vi "time_lua.vi"(5 "LuaVIEW reference":T1) -> (15 "error out":errorcluster)   [LabVIEW 2012]
doc: "Returns the time in seconds since the LabVIEW epoch (1-Jan-1904 00:00:00 GMT). When no parameter is specified, it returns the current time as obtained via \"Library Time.vi\", which exists to allow custom time sources. Its default implementation simply calls \"Get Date/Time In Seconds\" LabVIEW node, which in turn obtains its time from the system clock. Beware that the system clock has a platform dependent resolution and will drift unless corrected for, e.g. using the ntp protocol.\n\nWhen a parameter is specified, it should specify a date/time via a table with the following format: {year=<1904..2040>,month=<1..12>,day=<1..31>,[hour=<0..23>],[min=<0..59>],[sec=<0..59>]}. When the optional hour, min, or sec entries are omitted, they default to zero. The conversion to a time in seconds is performed using the standard \"Date/Time To Seconds\" LabVIEW function.\n\nBEWARE: the \"Date/Time To Seconds\" function yields a result that depends on the timezone and platform. Under Windows, the function corrects for daylight savings, when enabled. Under Linux, it does not, at least for LabVIEW versions 7.0 and 7.1. This is a bug: it yields a numerical time that can be one hour off when displayed via \"Format Date/Time String\".\nParameters:\n[tab:date]\nResults:\nnum:time\nErrors:\nInvalid date table.\nEntry out of range."
uses:
  typedefs/t_LuaVIEW Reference.ctl
  subvis/private/LuaVIEW Push (number).vi
  subvis/private/LuaVIEW Pull (flat data).vi
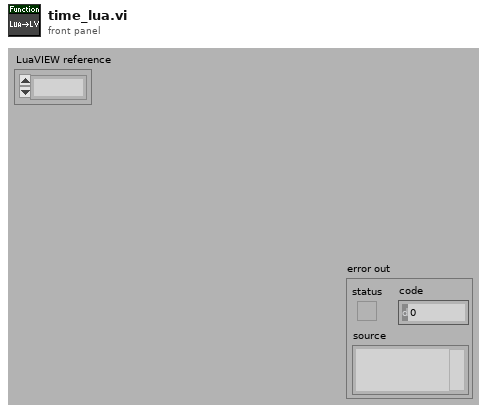
[diagram p1: front panel]
types:
  T1 = typedef "t_LuaVIEW Reference.ctl" = refnum<k1>
  T2 = cluster{"second":i32, "minute":i32, "hour":i32, "day of month":i32, "month":i32, "year":i32, "day of week":i32, "day of year":i32, "is DST":i32}
  T3 = cluster{"year":i32, "month":i32, "day":i32, "hour":i32, "min":i32, "sec":i32}
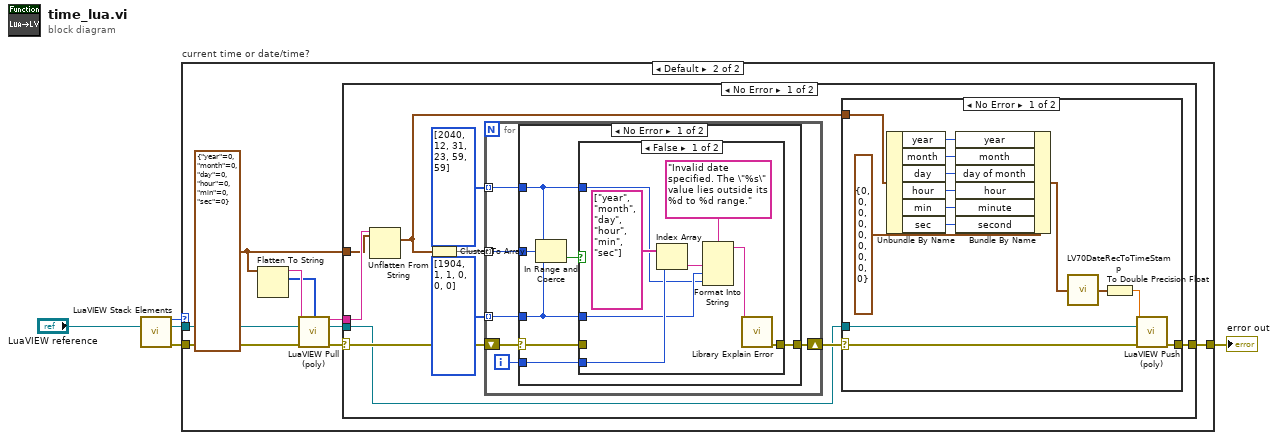
[diagram p0: block diagram]
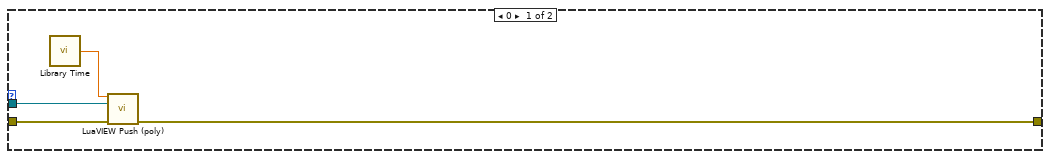
[diagram p2: hidden frame]
diagram:
  n1 = call "LuaVIEW Stack Elements.vi"("LuaVIEW reference in"="LuaVIEW reference") -> ("elements"=w3:i32, "LuaVIEW reference out"=w1:T1, "error out"=w2:errorcluster)  [unwired: 12 in]
  n2 = case "current time or date/time?" shown="Default" w3 {
    tunnel: [w6 w12] -> w5
    tunnel: w2 -> [w8 w10]
    tunnel: w1 -> [w7 w11]
    frame 0 {
      n3 = call "Library Time.vi"() -> ("time"=w9:dbl)  [unwired: 1 in]
      n4 = call-poly "LuaVIEW Push (poly).vi"("number"=w9, "LuaVIEW reference in"=w7, "error in (no error)"=w8) -> ("error out"=w6:errorcluster)  [unwired: 11 in, 1 out]
    }
    frame Default {
      w14 = T3 {"year"=0, "month"=0, "day"=0, "hour"=0, "min"=0, "sec"=0} ("date time rec")
      n5 = Flatten To String(anything=w14) -> (data string=w17:string, type string=w16:i16[])  [unwired: 3 in, 1 out]
      n6 = call-poly "LuaVIEW Pull (poly).vi"("default flat data"=w17, "type descriptor"=w16, "LuaVIEW reference in"=w11, "error in (no error)"=w10) -> ("flat data"=w15:string, "LuaVIEW reference out"=w18:T1, "error out"=w13:errorcluster)  [unwired: 9 in]
      n7 = case shown="No Error" w13 {
        selector: w13 -> [w25 w67]
        tunnel: w18 -> [w20 _]
        tunnel: [w28 w67] -> w12
        tunnel: w15 -> [w27 _]
        tunnel: w14 -> [w21 _]
        frame No Error {
          n8 = Unflatten From String(type=w21, binary string=w27) -> (value=w19:T3)  [unwired: 3 in, 2 out]
          n9 = Cluster To Array(cluster=w19) -> (array=w24:i32[])
          n10 = for {
            tunnel: w24 -> [w49] mode=indexing
            tunnel: i32[] [2040, 12, 31, 23, 59, 59] -> [w48] mode=indexing
            tunnel: i32[] [1904, 1, 1, 0, 0, 0] -> [w47] mode=indexing
            shift-right: [w45] -> w22
            shift-left: w25 -> [w46]
            i -> [w44]
            n11 = case shown="No Error" w46 {
              selector: w46 -> [w51 w66]
              tunnel: w49 -> [w56 _]
              tunnel: w48 -> [w54 _]
              tunnel: w47 -> [w53 _]
              tunnel: [w50 w66] -> w45
              tunnel: w44 -> [w52 _]
              frame No Error {
                n12 = In Range and Coerce(upper limit=w54, x=w56, lower limit=w53) -> (In Range?=w55:bool)  [unwired: 1 out]
                n13 = case shown="False" w55 {
                  tunnel: w54 -> [w57 _]
                  tunnel: w53 -> [w58 _]
                  tunnel: w52 -> [w63 _]
                  tunnel: w51 -> [_ w65]
                  tunnel: [w64 w65] -> w50
                  frame False {
                    n14 = Index Array(array=string[] ["year", "month", "day", "hour", "min", "sec"], index=w63) -> (element=w60:string)
                    n15 = Format Into String(format string="Invalid date specified. The \"%s\" value lies outside its %d to %d range.", w60, w58, w57) -> (resulting string=w59:string)  [unwired: 2 in, 1 out]
                    n16 = call "Library Explain Error.vi"("explanation prefix (none)"=w59) -> ("explained error"=w64:errorcluster)  [unwired: 14 in]
                  }
                  frame True {
                  }
                }
              }
              frame Error {
              }
            }
          }
          n17 = case shown="No Error" w22 {
            selector: w22 -> [w39 w43]
            tunnel: [w42 w43] -> w28
            tunnel: w19 -> [w38 _]
            tunnel: w20 -> [w29 _]
            frame No Error {
              n18 = Unbundle By Name(w38) -> ("year"=w30:i32, "month"=w31:i32, "day"=w32:i32, "hour"=w33:i32, "min"=w34:i32, "sec"=w35:i32)
              n19 = Bundle By Name(cluster=T2 {"second"=0, "minute"=0, "hour"=0, "day of month"=0, "month"=0, "year"=0, "day of week"=0, "day of year"=0, "is DST"=0} ("date time rec"), "year"=w30, "month"=w31, "day of month"=w32, "hour"=w33, "minute"=w34, "second"=w35) -> (w36:T2)
              n20 = call <vilib>:"LV70DateRecToTimeStamp.vi"("date time rec"=w36) -> ("Time Stamp"=w41:timestamp)
              n21 = To Double Precision Float(number=w41) -> (double precision float=w40:dbl)
              n22 = call-poly "LuaVIEW Push (poly).vi"("number"=w40, "LuaVIEW reference in"=w29, "error in (no error)"=w39) -> ("error out"=w42:errorcluster)  [unwired: 11 in, 1 out]
            }
            frame Error {
            }
          }
        }
        frame Error {
        }
      }
    }
  }
  "error out" <- w5
